vi "gxml_GetTypeDefVersion.vi"(7 "Version Tag Name":string, 8 "error in":errorcluster, 10 "XML String In":string) -> (0 "error out":errorcluster, 2 "XML String Out":string, 3 "Version String":string)   [LabVIEW 2009]
doc: "This VI looks for a version tag name inside the XML string and return the version as a string.\n\n\"gxml_Generator.vi\" has optional inputs which will add a tagged version string to the XML string. This is useful so that the consumer application can determine which type def to use for parsing and how to update data from old XML files to the current version."
uses:
  <vilib>/regexp/Match Regular Expression.xnode
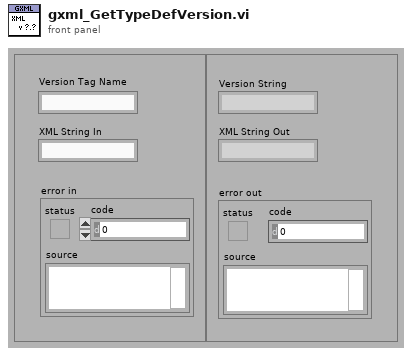
[diagram p1: front panel]
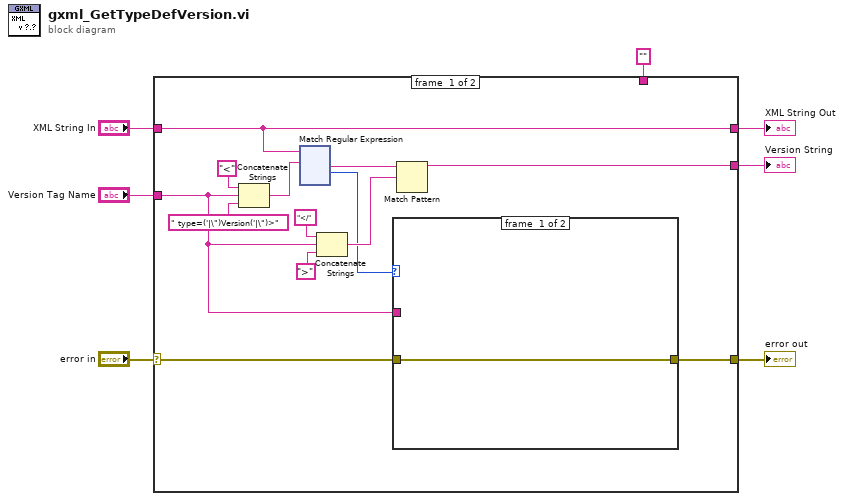
[diagram p0: block diagram]
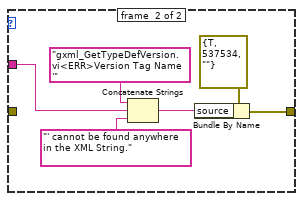
[diagram p2: hidden frame]
diagram:
  n1 = case shown="No Error" "error in" {
    selector: "error in" -> [w19 w137]
    tunnel: "XML String In" -> [w9 w136]
    tunnel: "Version Tag Name" -> [w17 _]
    tunnel: [w20 w135] -> w5
    tunnel: [w18 w137] -> w4
    tunnel: "" ("XML String In") -> [_ w135]
    tunnel: [w9 w136] -> w1
    frame #0 {
      n2 = Concatenate Strings("<", w17, " type=('|\")Version('|\")>") -> (w15:string)
      n3 = xnode "Match Regular Expression"("input string"=w9, "regular expression"=w15) -> ("after match"=w14:string, "offset past match"=w8:i32)  [unwired: 4 in, 3 out]
      n4 = Concatenate Strings("</", w17, ">") -> (w12:string)
      n5 = case shown="-1" w8 {
        tunnel: w19 -> [w128 _]
        tunnel: [w128 w133] -> w18
        tunnel: w17 -> [_ w129]
        frame #0 {
        }
        frame #1 {
          n6 = Concatenate Strings("gxml_GetTypeDefVersion.vi<ERR>Version Tag Name '", w129, "' cannot be found anywhere in the XML String.") -> (w130:string)
          n7 = Bundle By Name(cluster=errorcluster {"status"=TRUE, "code"=537534, "source"=""} ("error in"), "source"=w130) -> (w133:errorcluster)
        }
      }
      n8 = Match Pattern(string=w14, regular expression=w12) -> (before substring=w20:string)  [unwired: 1 in, 3 out]
    }
    frame #1 {
    }
  }
  "Version String" <- w5
  "error out" <- w4
  "XML String Out" <- w1
